vi "P3060_关闭设备.vi"(8 "error in (no error)":errorcluster caption="错误输入（无错误）", 11 "句柄输入":i32) -> (0 "error out":errorcluster caption="错误输出")   [LabVIEW 2012]
doc: "关闭板卡"
uses:
  _SubVI/dll/Release/P3060.dll
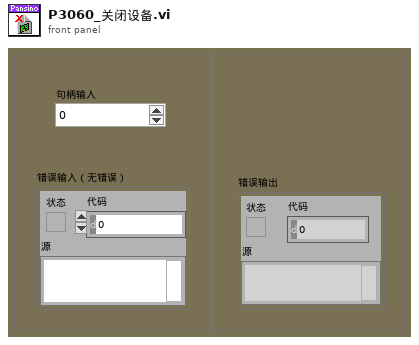
[diagram p1: front panel]
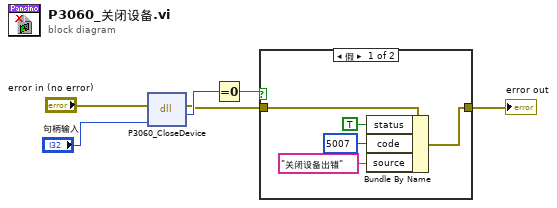
[diagram p0: block diagram]
diagram:
  n1 = dll-call lib="C:/PLC_simulation/2014.2.25PLC_NEW/PLC_NEW/P3060NEW/_SubVI/dll/Release/P3060.dll" fn="P3060_CloseDevice"(error in="error in (no error)", "hDev"="句柄输入") -> (error out=w1:errorcluster, "hDevOut"=w3:i32)  [unwired: 3 in, 1 out]
  n2 = Equal To 0?(x=w3) -> (x = 0?=w2:bool)
  n3 = case shown="假" w2 {
    tunnel: [w10 w12] -> w5
    tunnel: w1 -> [w11 w12]
    frame False {
      n4 = Bundle By Name(cluster=w11, "status"=TRUE, "code"=5007, "source"="关闭设备出错") -> (w10:errorcluster)
    }
    frame True {
    }
  }
  "error out" <- w5
